vi "DVR Access.vi"(0 "Input":dbl, 2 "Stop":bool, 11 "Error In":errorcluster) -> (4 "Output":dbl, 15 "Error Out":errorcluster)   [LabVIEW 2023]
doc: "This VI creates a DVR and passes it to 4 loops and performs operation in 3 loops and read the data value in the 4th loop."
panel:
  # "Instruction:\n\n1. Run the VI.\n2. Specify the input.\n3. Observe the output in the indicator.\n4. Press stop to stop running the VI.\n5. Open the block diagram and make changes in the wait time, settings of the in place element to observe the behaviour of DVRs."
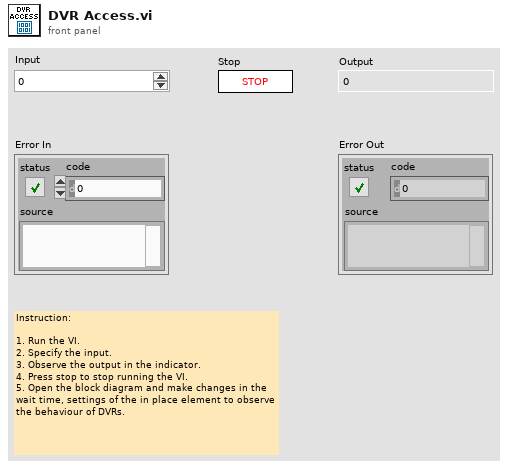
[diagram p1: front panel]
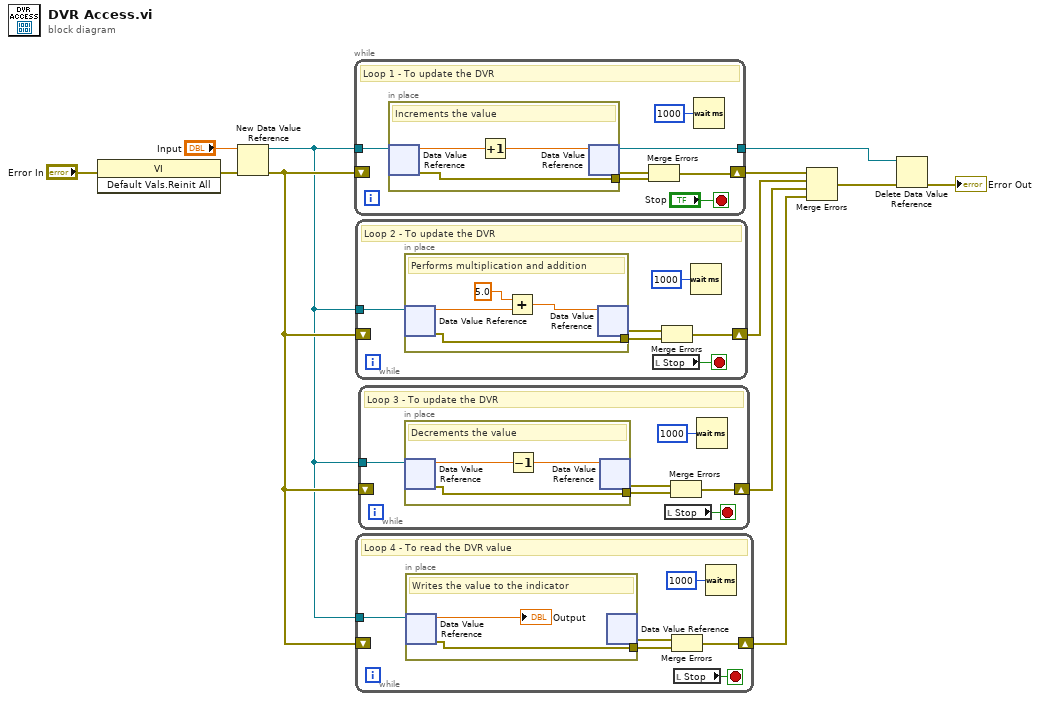
[diagram p0: block diagram]
diagram:
  n1 = invoke class="VI" method="Default Vals.Reinit All"(error in="Error In") -> (error out=w1:errorcluster)  [unwired: 2 in, 2 out]
  n2 = New Data Value Reference(data value="Input", error in=w1) -> (data value reference=w2:refnum<data-value>, error out=w5:errorcluster)
  n3 = while {
    shift-right: [w13] -> w11
    shift-left: w5 -> [_]
    tunnel: w2 -> [w18]
    tunnel: [w17] -> w6
    stop <- "Stop" stop-if-true
    # "Loop 1 - To update the DVR"
    n4 = in-place {
      in-place-border: [w20] -> w14
      # "Increments the value"
      n5 = in-place-dvr #1(w18) -> (w21:dbl, w20:errorcluster)
      n6 = Increment(x=w21) -> (x+1=w22:dbl)
      n7 = in-place-dvr #1(w22) -> (w17:refnum<data-value>, w15:errorcluster)
    }
    n8 = Merge Errors(w15, w14) -> (w13:errorcluster)
    n9 = Wait (ms)(milliseconds to wait=u32 1000) -> ()  [unwired: 1 out]
  }
  n10 = while {
    shift-right: [w24] -> w3
    shift-left: w5 -> [_]
    tunnel: w2 -> [w27]
    stop <- w26 stop-if-true
    # "Loop 2 - To update the DVR"
    n11 = in-place {
      in-place-border: [w29] -> w23
      # "Performs multiplication and addition"
      n12 = in-place-dvr #2(w27) -> (w31:dbl, w29:errorcluster)
      n13 = Add(x=5.0, y=w31) -> (x+y=w30:dbl)
      n14 = in-place-dvr #2(w30) -> (w25:errorcluster)  [unwired: 1 out]
    }
    n15 = local read "Stop"() -> (w26:bool)
    n16 = Merge Errors(w25, w23) -> (w24:errorcluster)
    n17 = Wait (ms)(milliseconds to wait=u32 1000) -> ()  [unwired: 1 out]
  }
  n18 = while {
    shift-right: [w33] -> w8
    shift-left: w5 -> [_]
    tunnel: w2 -> [w38]
    stop <- w36 stop-if-true
    # "Loop 4 - To read the DVR value"
    n19 = in-place {
      in-place-border: [w40] -> w34
      # "Writes the value to the indicator"
      n20 = in-place-dvr #3(w38) -> (→"Output":dbl, w40:errorcluster)
      n21 = in-place-dvr #3() -> (w35:errorcluster)  [unwired: 1 in, 1 out]
    }
    n22 = Merge Errors(w35, w34) -> (w33:errorcluster)
    n23 = local read "Stop"() -> (w36:bool)
    n24 = Wait (ms)(milliseconds to wait=u32 1000) -> ()  [unwired: 1 out]
  }
  n25 = while {
    shift-right: [w41] -> w4
    shift-left: w5 -> [_]
    tunnel: w2 -> [w46]
    stop <- w44 stop-if-true
    # "Loop 3 - To update the DVR"
    n26 = in-place {
      in-place-border: [w47] -> w42
      # "Decrements the value"
      n27 = in-place-dvr #4(w46) -> (w49:dbl, w47:errorcluster)
      n28 = Decrement(x=w49) -> (x-1=w48:dbl)
      n29 = in-place-dvr #4(w48) -> (w43:errorcluster)  [unwired: 1 out]
    }
    n30 = local read "Stop"() -> (w44:bool)
    n31 = Merge Errors(w43, w42) -> (w41:errorcluster)
    n32 = Wait (ms)(milliseconds to wait=u32 1000) -> ()  [unwired: 1 out]
  }
  n33 = Merge Errors(w11, w3, w4, w8) -> (w9:errorcluster)
  n34 = Delete Data Value Reference(data value reference=w6, error in=w9) -> (error out=→"Error Out":errorcluster)  [unwired: 1 out]
